vi "Keyence I32 to U8 array.vi"(11 "Numeric":i32) -> (3 "Array":u8[](array[numeric]))   [LabVIEW 2018]
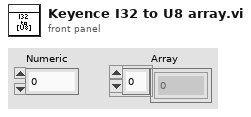
[diagram p1: front panel]
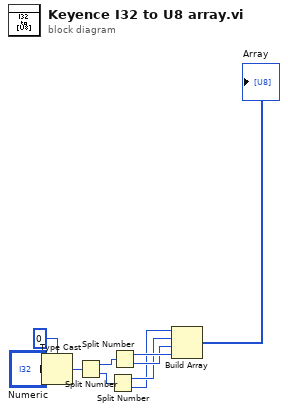
[diagram p0: block diagram]
diagram:
  n1 = Type Cast(type=u32 0 ("(hi.lo)"), x="Numeric") -> (*(type *) &x=w3:u32)
  n2 = Split Number(x=w3) -> (hi(x)=w4:u16, lo(x)=w5:u16)
  n3 = Split Number(x=w5) -> (hi(x)=w7:u8, lo(x)=w6:u8)
  n4 = Split Number(x=w4) -> (hi(x)=w9:u8, lo(x)=w8:u8)
  n5 = Build Array(w6, w7, w8, w9) -> (→"Array":u8[])
